vi "Plotter FGV Data.vi"(8 "error in":errorcluster, 10 "Function":enum16{"Read", "Write", "Clear"}(ring), 11 "Data in":dbl[][](array[numeric])) -> (0 "error out":errorcluster, 3 "Data out":dbl[][](array[numeric]))   [LabVIEW 2013]
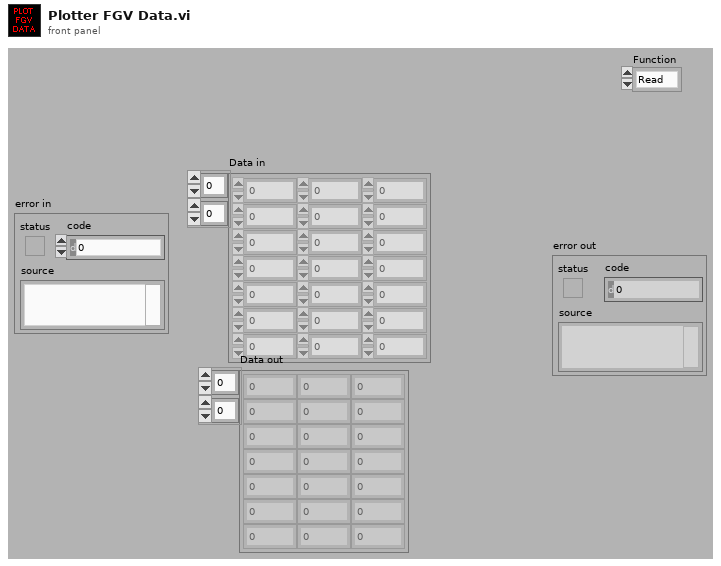
[diagram p1: front panel]
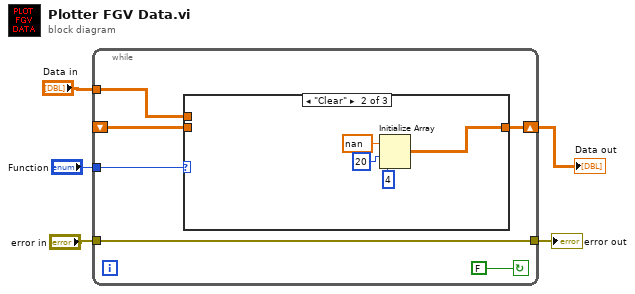
[diagram p0: block diagram]
diagram:
  n1 = while {
    shift-right: [w9] -> w2
    shift-left: _ -> [w8]
    tunnel: "Function" -> [w11]
    tunnel: "Data in" -> [w10]
    tunnel: "error in" -> [w6]
    tunnel: [w6] -> w3
    stop <- FALSE continue-if-true
    n2 = case shown="\"Clear\"" w11 {
      tunnel: w10 -> [_ _ w17]
      tunnel: [w12 w13 w17] -> w9
      tunnel: w8 -> [w12 _ _]
      frame "Read", Default {
      }
      frame "Clear" {
        n3 = Initialize Array(nan ("element"), 20 ("dimension size"), 4 ("dimension size")) -> (w13:dbl[][])
      }
      frame "Write" {
      }
    }
  }
  "error out" <- w3
  "Data out" <- w2
